vi "RM.getNodeReservations.vi"(7 "Resource Type":T1, 8 "error in":errorcluster, 11 "Item Ref in":T2 format="%.0x") -> (0 "error out":errorcluster, 1 "clientGUIDs":string[](array[string]), 2 "names in bitfile":string[](array[string]), 3 "Item Ref out":T2 format="%.0x")   [LabVIEW 2016, in "FPGA Resource Manager.lvlib"]
uses:
  FPGA Resource Manager.lvlib
  <vilib>/NI Veristand/Custom Device API/Custom Device Item Ref.ctl
  RM.resourceType.ctl
  <vilib>/NI VeriStand/Custom Device API/Custom Device API.lvlib
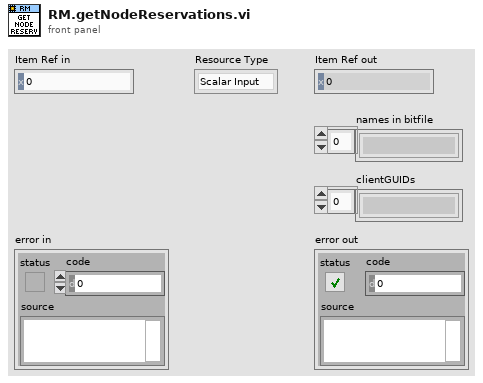
[diagram p1: front panel]
types:
  T1 = typedef "FPGA Resource Manager.lvlib/RM.resourceType.ctl" = enum16{"Scalar Input", "Scalar Output", "Waveform Input", "Waveform Output"}
  T2 = typedef "Custom Device API.lvlib/Custom Device Item Ref.ctl" = u64
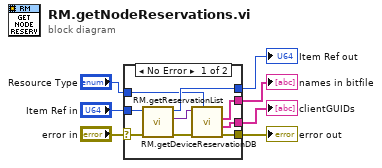
[diagram p0: block diagram]
diagram:
  n1 = case shown="No Error" "error in" {
    selector: "error in" -> [w10 w17]
    tunnel: "Item Ref in" -> [w15 w18]
    tunnel: [w14 w18] -> w6
    tunnel: [w12 _] -> w5
    tunnel: [w11 _] -> w4
    tunnel: [w9 w17] -> w2
    tunnel: "Resource Type" -> [w8 _]
    frame No Error {
      n2 = call "RM.getDeviceReservationDB.vi"("error in"=w10, "Item Ref in"=w15) -> ("error out"=w13:errorcluster, "reservation DB out"=w16:variant, "Item Ref out"=w14:T2)  [unwired: 6 in, 1 out]
      n3 = call "RM.getReservationList.vi"("Resource Type"=w8, "error in"=w13, "reservation DB in"=w16) -> ("error out"=w9:errorcluster, "clientGUIDs"=w11:string[], "names in bitfile"=w12:string[])  [unwired: 5 in, 1 out]
    }
    frame Error {
    }
  }
  "Item Ref out" <- w6
  "names in bitfile" <- w5
  "clientGUIDs" <- w4
  "error out" <- w2
